vi "Update Time Display Objects.vi"(8 "Error In":errorcluster, 11 "Display Manager In":refnum<class "Display Manager.lvclass">) -> (0 "Error Out":errorcluster, 3 "Display Manager Out":refnum<class "Display Manager.lvclass">)   [LabVIEW 2021, in "Display Manager.lvclass"]
uses:
  Display Manager.lvclass
  <vilib>/Memosfet/myRIO-Neopixel/RT/String/String.lvclass
  Accessors/Display/Get Display.vi
  <vilib>/Memosfet/myRIO-Neopixel/RT/Display/Display.lvclass
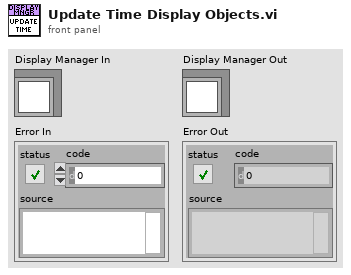
[diagram p1: front panel]
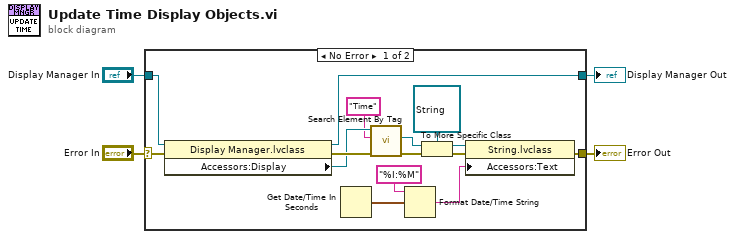
[diagram p0: block diagram]
diagram:
  n1 = case shown="No Error" "Error In" {
    selector: "Error In" -> [w18 w21]
    tunnel: [w16 w21] -> w3
    tunnel: "Display Manager In" -> [w19 w20]
    tunnel: [w17 w20] -> w1
    frame No Error {
      n2 = property class="Display Manager.lvclass"(reference=w19, error in=w18) -> (reference out=w17:refnum<class "Display Manager.lvclass">, error out=w9:errorcluster, "Accessors:Display"=w6:refnum<class "Display.lvclass">)
      n3 = Get Date/Time In Seconds() -> (seconds since 1Jan1904=w11:timestamp)
      n4 = call <vilib>:"Search Element By Tag.vi"("Error In"=w9, "Element Tag"="Time" ("Tag"), "Display In"=w6) -> ("Error Out"=w7:errorcluster, "Display Element"=w8:refnum<class "Display Element.lvclass">)  [unwired: 5 in, 2 out]
      n5 = Format Date/Time String(time format string (%c)="%I:%M", seconds (now)=w11) -> (date/time string=w10:string)  [unwired: 1 in]
      n6 = To More Specific Class(target class=refnum<class "String.lvclass"> refnum ("Pixel In"), reference=w8, error in=w7) -> (specific class reference=w14:refnum<class "String.lvclass">, error out=w13:errorcluster)
      n7 = property class="String.lvclass"(reference=w14, error in=w13, "Accessors:Text"=w10) -> (error out=w16:errorcluster)  [unwired: 1 out]
    }
    frame Error {
    }
  }
  "Display Manager Out" <- w1
  "Error Out" <- w3
